vi "UDP Experiment.vi"(7 "stop":bool, 10 "Host Port":u16=55555) -> (0 "Source Port":u16, 1 "Source Address":u32, 3 "data out":string, 4 "Time Since Last Packet":u32)   [LabVIEW 2013]
panel:
  out "Iteration":i32
  out "Length":i32
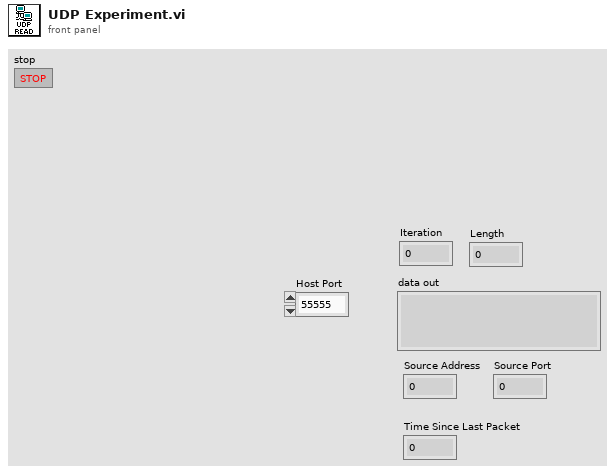
[diagram p1: front panel]
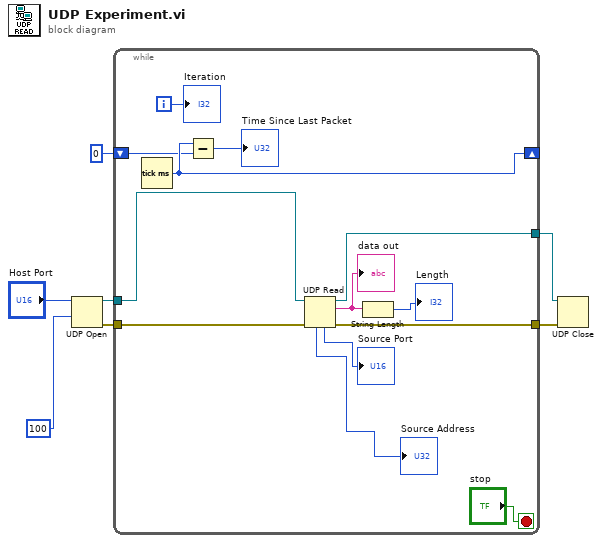
[diagram p0: block diagram]
diagram:
  n1 = UDP Open(9:100 ("timeout ms (25000)"), 11:"Host Port") -> (port=w3:refnum<k16>, 0:w4:errorcluster)  [unwired: 3 in, 1 out]
  n2 = while {
    tunnel: w3 -> [w20]
    tunnel: w4 -> [w19]
    tunnel: [w18] -> w6
    tunnel: [w17] -> w5
    shift-right: [w10] -> _
    shift-left: u32 0 ("millisecond timer value") -> [w9]
    i -> [w11]
    stop <- "stop" stop-if-true
    n3 = Tick Count (ms)() -> (millisecond timer value=w10:u32)
    n4 = Subtract(x=w10, y=w9) -> (x-y=→"Time Since Last Packet":u32)
    n5 = UDP Read(connection ID=w20, 8:w19) -> (data out=w13:string, error out=w18:errorcluster, 3:w17:refnum<k16>, 4:→"Source Port":u16, 6:→"Source Address":u32)  [unwired: 2 in]
    "data out" <- w13
    n6 = String Length(string=w13) -> (length=→"Length":i32)
    "Iteration" <- w11
  }
  n7 = UDP Close(connection ID=w5, 8:w6) -> ()  [unwired: 2 out]
